vi "SVPO Limit Testing (1 Ch) (SGL Array) with IC.vi"(7 "reset? (F)":bool, 8 "initial conditions":T1={"upper limit clearance"=inf, "lower limit clearance"=inf, "test passed?"=TRUE, "block passed?"=FALSE}, 9 "lower limit":sgl=-inf format="%.2f", 10 "upper limit":sgl=inf format="%.2f", 11 "signal in":sgl[](array[numeric])) -> (0 "final conditions":T1, 1 "lower limit clearance":sgl format="%.6f", 2 "upper limit clearance":sgl format="%.6f", 3 "test passed?":bool)   [LabVIEW 2017, in "SoundVib_LimitTest.lvlib"]
doc: "Performs limit testing on single-precision waveforms, single-precision scaled arrays, or double-precision scalar measurements. You can specify an upper and lower boundary of the envelope to define a pass range. This VI uses the defined pass range to test the input signal. VI outputs apply to all the tests since the last VI reset. Use this VI on embedded targets that have limited computational resources. Wire data to the <B>value in</B> input to determine the polymorphic instance to use or manually select the instance."
uses:
  <vilib>/addons/Sound and Vibration/svt_Limit Test/SoundVib_LimitTest.lvlib
  <vilib>/addons/_NISVFA/_Shared subVIs/Controls/svc_SGL Limit State.ctl
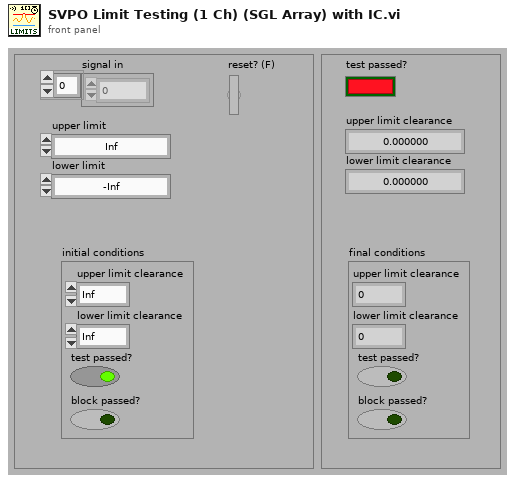
[diagram p1: front panel]
types:
  T1 = typedef "svc_SGL Limit State.ctl" = cluster{"upper limit clearance":sgl, "lower limit clearance":sgl, "test passed?":bool, "block passed?":bool}
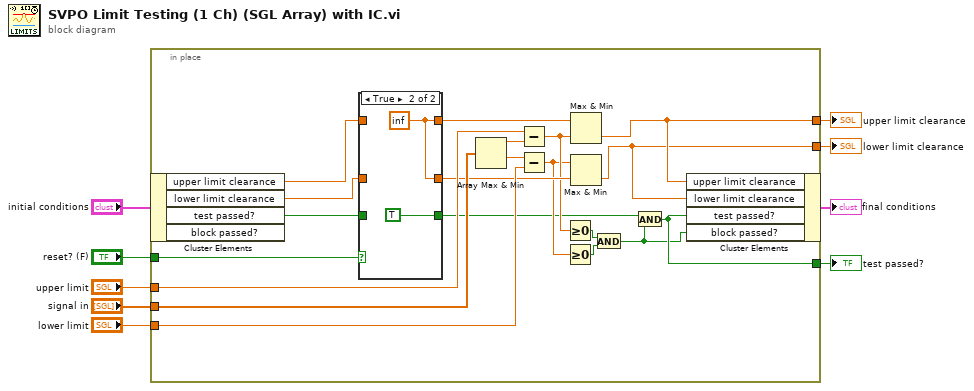
[diagram p0: block diagram]
diagram:
  n1 = in-place {
    in-place-border: "upper limit" -> [w29]
    in-place-border: "lower limit" -> [w28]
    in-place-border: [w16] -> w7
    in-place-border: [w15] -> w6
    in-place-border: "signal in" -> [w27]
    in-place-border: [w11] -> w4
    in-place-border: "reset? (F)" -> [w26]
    n2 = in-place-cluster #1("initial conditions") -> ("upper limit clearance"=w19:sgl, "lower limit clearance"=w17:sgl, "test passed?"=w18:bool)  [unwired: 1 out]
    n3 = case shown="True" w26 {
      tunnel: w19 -> [w32 _]
      tunnel: [w32 w33] -> w25
      tunnel: w17 -> [w31 _]
      tunnel: [w31 w33] -> w24
      tunnel: w18 -> [w30 _]
      tunnel: [w30 TRUE] -> w12
      frame False {
      }
      frame True {
        w33 = sgl inf
      }
    }
    n4 = Array Max & Min(array=w27) -> (max value=w23:sgl, min value=w22:sgl)  [unwired: 2 out]
    n5 = Subtract(x=w29, y=w23) -> (x-y=w21:sgl)
    n6 = Subtract(x=w22, y=w28) -> (x-y=w20:sgl)
    n7 = Greater Or Equal To 0?(x=w21) -> (x >= 0?=w13:bool)
    n8 = Greater Or Equal To 0?(x=w20) -> (x >= 0?=w14:bool)
    n9 = Max & Min(x=w25, y=w21) -> (min(x,y)=w16:sgl)  [unwired: 1 out]
    n10 = Max & Min(x=w20, y=w24) -> (min(x,y)=w15:sgl)  [unwired: 1 out]
    n11 = And(x=w13, y=w14) -> (x .and. y?=w10:bool)
    n12 = And(x=w12, y=w10) -> (x .and. y?=w11:bool)
    n13 = in-place-cluster #1("upper limit clearance"=w16, "lower limit clearance"=w15, "test passed?"=w11, "block passed?"=w10) -> (→"final conditions":T1)
  }
  "test passed?" <- w4
  "upper limit clearance" <- w7
  "lower limit clearance" <- w6
